vi "FIFO.vi"(0 "数值":dbl, 1 "元素大小":u32, 2 "启用":bool, 3 "初始化":bool) -> (4 "数组":dbl[](array[numeric]))   [LabVIEW 2016, in "多参数状态显示.xctl"]
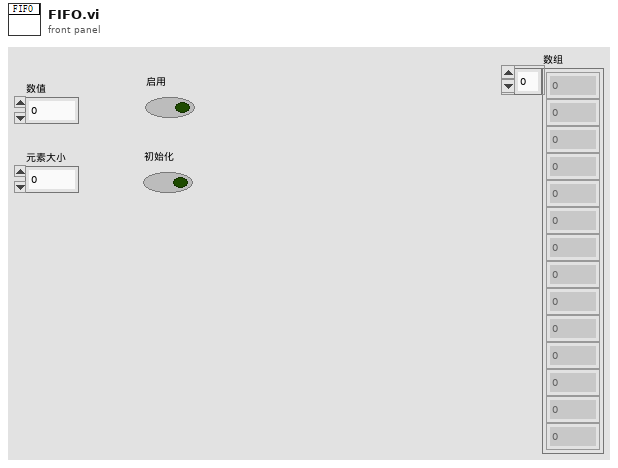
[diagram p1: front panel]
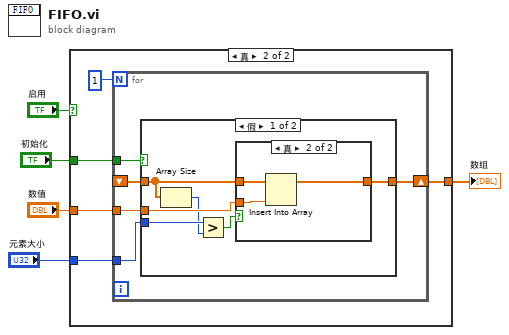
[diagram p0: block diagram]
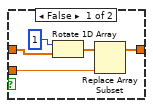
[diagram p3: hidden frame]
diagram:
  n1 = case shown="真" "启用" {
    tunnel: "数值" -> [_ w10]
    tunnel: "元素大小" -> [_ w9]
    tunnel: [_ w8] -> w3
    tunnel: "初始化" -> [_ w6]
    frame False {
    }
    frame True {
      n2 = for {
        N: 1 -> [_]
        tunnel: w10 -> [w15]
        shift-right: [w14] -> w8
        shift-left: _ -> [w13]
        tunnel: w9 -> [w12]
        tunnel: w6 -> [w11]
        n3 = case shown="假" w11 {
          tunnel: w15 -> [w21 _]
          tunnel: [w20 _] -> w14
          tunnel: w13 -> [w19 _]
          tunnel: w12 -> [w18 _]
          frame False {
            n4 = Array Size(array=w19) -> (size(s)=w17:i32)
            n5 = Greater?(x=w18, y=w17) -> (0:w16:bool)
            n6 = case shown="真" w16 {
              tunnel: w21 -> [w25 w29]
              tunnel: [w23 w28] -> w20
              tunnel: w19 -> [w26 w27]
              frame False {
                n7 = Rotate 1D Array(1:w26, 2:1 ("n")) -> (0:w24:dbl[])
                n8 = Replace Array Subset(array=w24, new element=w25) -> (w23:dbl[])  [unwired: 1 in]
              }
              frame True {
                n9 = Insert Into Array(array=w27, new element=w29) -> (w28:dbl[])  [unwired: 1 in]
              }
            }
          }
          frame True {
          }
        }
      }
    }
  }
  "数组" <- w3
